vi "Construct Command - LoadFile.vi"(8 "error in (no error)":errorcluster, 10 "LoadFile Configuration":T1) -> (0 "error out":errorcluster, 2 "Command":string)   [LabVIEW 2016, in "JLink Commander.lvlib"]
doc: "Construct a LoadFile command which programs a given data file. For .bin files, a location has to be specified. By default also performs a verification of programmed data. Currently supported data files are: .bin, .elf, .hex, .mot, .s, .s19, .s37, .srec."
uses:
  JLink Commander.lvlib
  Type Definitions/LoadFile Configuration.ctl
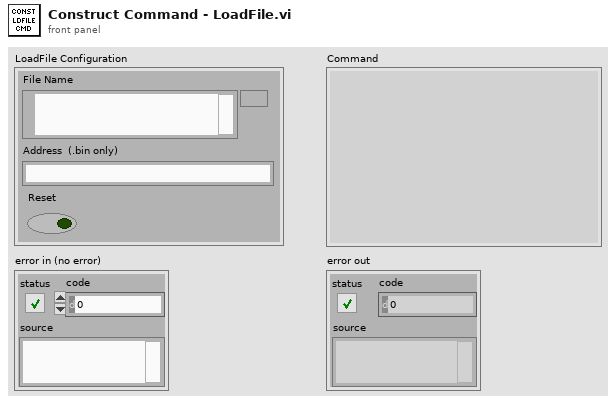
[diagram p1: front panel]
types:
  T1 = typedef "JLink Commander.lvlib/LoadFile Configuration.ctl" = cluster{"File Name":path, "Address":string, "Reset":bool}
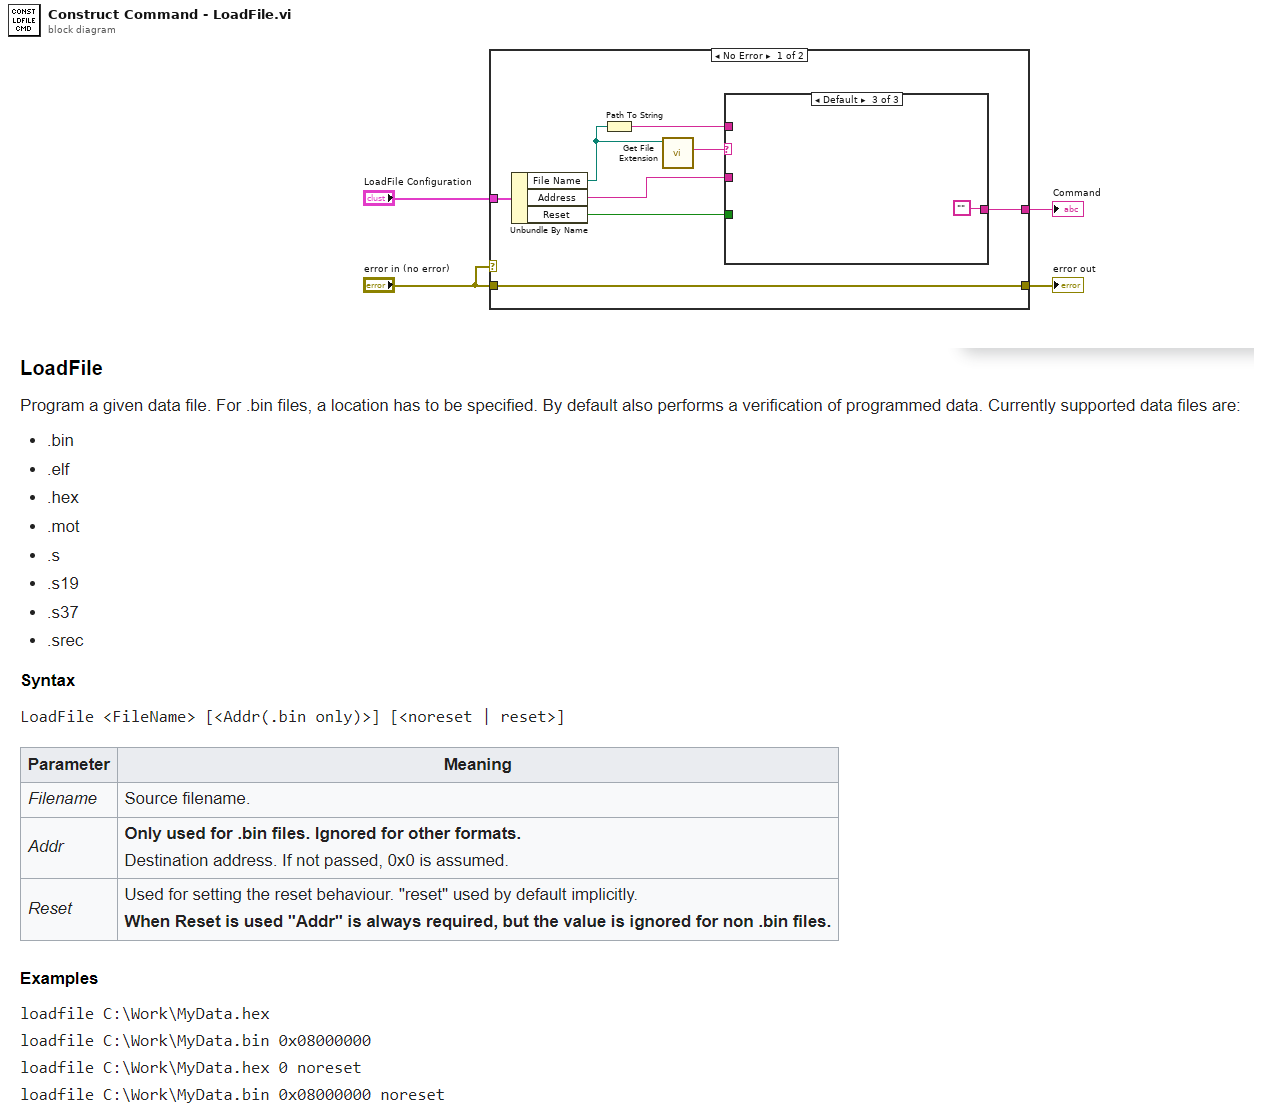
[diagram p0: block diagram]
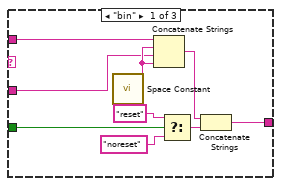
[diagram p2: hidden frame]
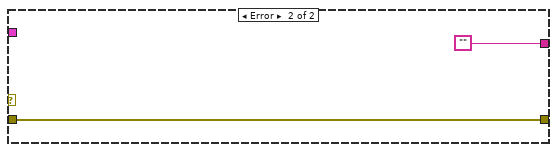
[diagram p4: hidden frame]
diagram:
  n1 = case shown="No Error" "error in (no error)" {
    tunnel: "LoadFile Configuration" -> [w9 _]
    tunnel: [w8 ""] -> w3
    tunnel: [w7 w24] -> w2
    tunnel: "error in (no error)" -> [w7 w24]
    frame No Error {
      n2 = Unbundle By Name(w9) -> ("File Name"=w6:path, "Address"=w11:string, "Reset"=w10:bool)
      n3 = Path To String(path=w6) -> (string=w12:string)
      n4 = call <vilib>:"Get File Extension.vi"("file"=w6) -> ("lowercase file extension"=w5:string)  [unwired: 6 in, 4 out]
      n5 = case shown="Default" w5 {
        tunnel: w12 -> [w19 w22 _]
        tunnel: w11 -> [w13 _ _]
        tunnel: w10 -> [w18 _ _]
        tunnel: [w17 w22 ""] -> w8
        frame "bin" {
          n6 = call <vilib>:"Space Constant.vi"() -> ("String"=w20:string)
          n7 = Concatenate Strings(w19, w20, w13, w20) -> (w21:string)
          n8 = Select(t="reset", s=w18, f="noreset") -> (s? t:f=w16:string)
          n9 = Concatenate Strings(w21, w16) -> (w17:string)
        }
        frame "hex" {
        }
        frame Default {
        }
      }
    }
    frame Error {
    }
  }
  "Command" <- w3
  "error out" <- w2
